vi "GlobalTemp1.vi"() -> ()   [LabVIEW 2024]
panel:
  out "Temp1":dbl
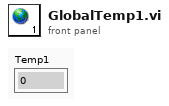
[diagram p1: front panel]
diagram:
